vi "Make Node Name Unique.vi"(9 "New Node Name":string, 10 "Parent Path":string, 11 "Tree Map In":T1) -> (2 "Node Path":string)   [LabVIEW 2020, in "Tree Map.lvlib"]
doc: "<b>Author:</b> Piotr Kruczkowski <PrimaryKey>\n<b>License:</b> NewBSD\n\nCopyright (c) 2019, National Instruments\nAll rights reserved.\n\nRedistribution and use in source and binary forms, with or without\nmodification, are permitted provided that the following conditions are met:\n1. Redistributions of source code must retain the above copyright\n notice, this list of conditions and the following disclaimer.\n2. Redistributions in binary form must reproduce the above copyright\n notice, this list of conditions and the following disclaimer in the\n documentation and/or other materials provided with the distribution.\n3. Neither the name of National Instruments nor the\n names of its contributors may be used to endorse or promote products\n derived from this software without specific prior written permission.\n\nTHIS SOFTWARE IS PROVIDED BY National Instruments ''AS IS'' AND ANY\nEXPRESS OR IMPLIED WARRANTIES, INCLUDING, BUT NOT LIMITED TO, THE IMPLIED\nWARRANTIES OF MERCHANTABILITY AND FITNESS FOR A PARTICULAR PURPOSE ARE\nDISCLAIMED. IN NO EVENT SHALL National Instruments BE LIABLE FOR ANY\nDIRECT, INDIRECT, INCIDENTAL, SPECIAL, EXEMPLARY, OR CONSEQUENTIAL DAMAGES\n(INCLUDING, BUT NOT LIMITED TO, PROCUREMENT OF SUBSTITUTE GOODS OR SERVICES;\nLOSS OF USE, DATA, OR PROFITS; OR BUSINESS INTERRUPTION) HOWEVER CAUSED AND\nON ANY THEORY OF LIABILITY, WHETHER IN CONTRACT, STRICT LIABILITY, OR TORT\n(INCLUDING NEGLIGENCE OR OTHERWISE) ARISING IN ANY WAY OUT OF THE USE OF THIS\nSOFTWARE, EVEN IF ADVISED OF THE POSSIBILITY OF SUCH DAMAGE."
uses:
  Tree Map.lvlib
  Tree Map Data.ctl
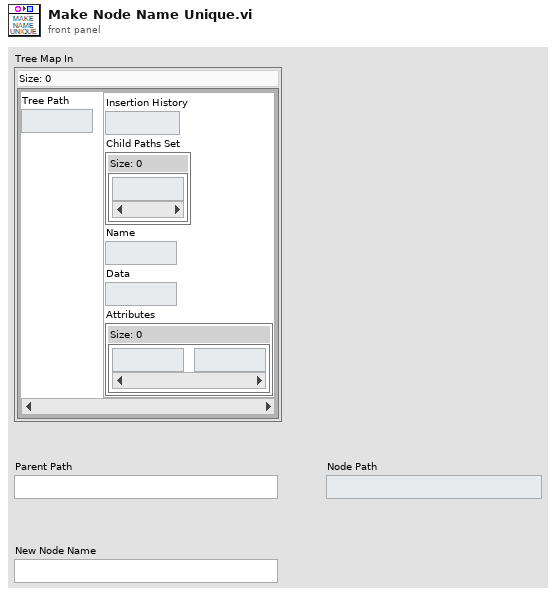
[diagram p1: front panel]
types:
  T1 = typedef "Tree Map.lvlib/Tree Map Data.ctl" = map{string, cluster{"Insertion History":i32, "Child Paths Set":set{string}, "Name":string, "Data":string, "Attributes":map{string, string}}}
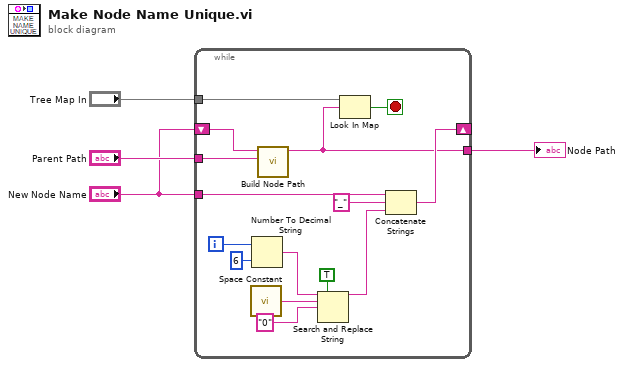
[diagram p0: block diagram]
diagram:
  n1 = while {
    tunnel: "Tree Map In" -> [w19]
    tunnel: "Parent Path" -> [w17]
    shift-right: [w14] -> _
    shift-left: "New Node Name" -> [w16]
    tunnel: [w13] -> w4
    tunnel: "New Node Name" -> [w12]
    i -> [w9]
    stop <- w18 stop-if-true
    n2 = call <vilib>:"Space Constant.vi"() -> ("String"=w7:string)
    n3 = Number To Decimal String(number=w9, width (-)=i16 6) -> (decimal integer string=w8:string)
    n4 = call "Build Node Path.vi"("Parent Path"=w17, "Node Name"=w16) -> ("Node Path"=w13:string)  [unwired: 9 in]
    n5 = Search and Replace String(replace all?=TRUE ("replace all? (F)"), input string=w8, search string=w7, replace string="0" ("replace string (\"\")")) -> (result string=w5:string)  [unwired: 4 in, 3 out]
    n6 = Look In Map(map=w19, key=w13) -> (key not found?=w18:bool)  [unwired: 1 in, 1 out]
    n7 = Concatenate Strings(w12, "_" ("string"), w5) -> (w14:string)
  }
  "Node Path" <- w4
